vi "Data Server Find Indexes from Variable Names.vi"(8 "Comand string":string, 11 "Variable names":string[](array[string])) -> (0 "Command error":bool, 3 "Index array":i32[](array[numeric]))   [LabVIEW 2011, in "Data Server VIs.lvlib"]
uses:
  Data Server VIs.lvlib
panel:
  in  "Number of BPM":i32
  in  "comand string 2":string="ACH05AACH06ACH07AACH02ACH01B"
  in  "BPM names":string[](array[string])=["ACH01B", "ACH02", "ACH03B", "ACH04", "ACH05A", "ACH06", "ACH07A", "ACH07B", "ACH08"]
  out "Command error 2":bool
  out "Index array 2":i32[](array[numeric])
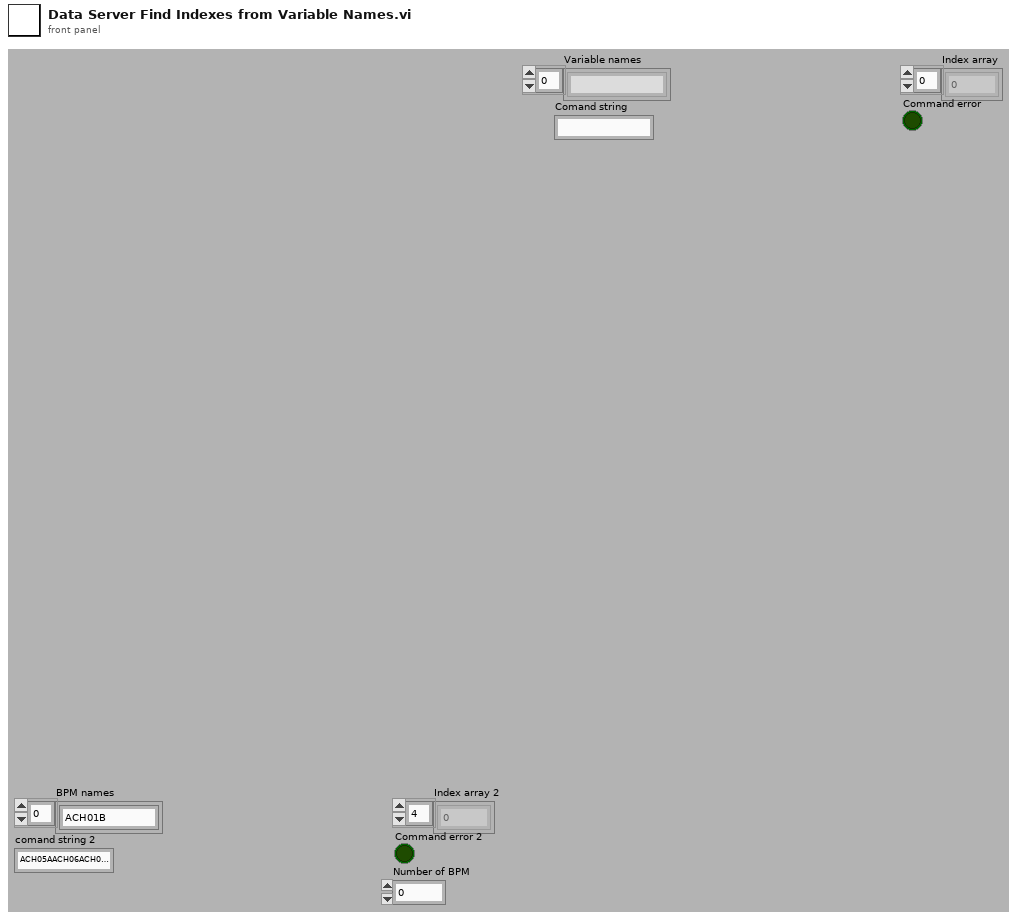
[diagram p1: front panel]
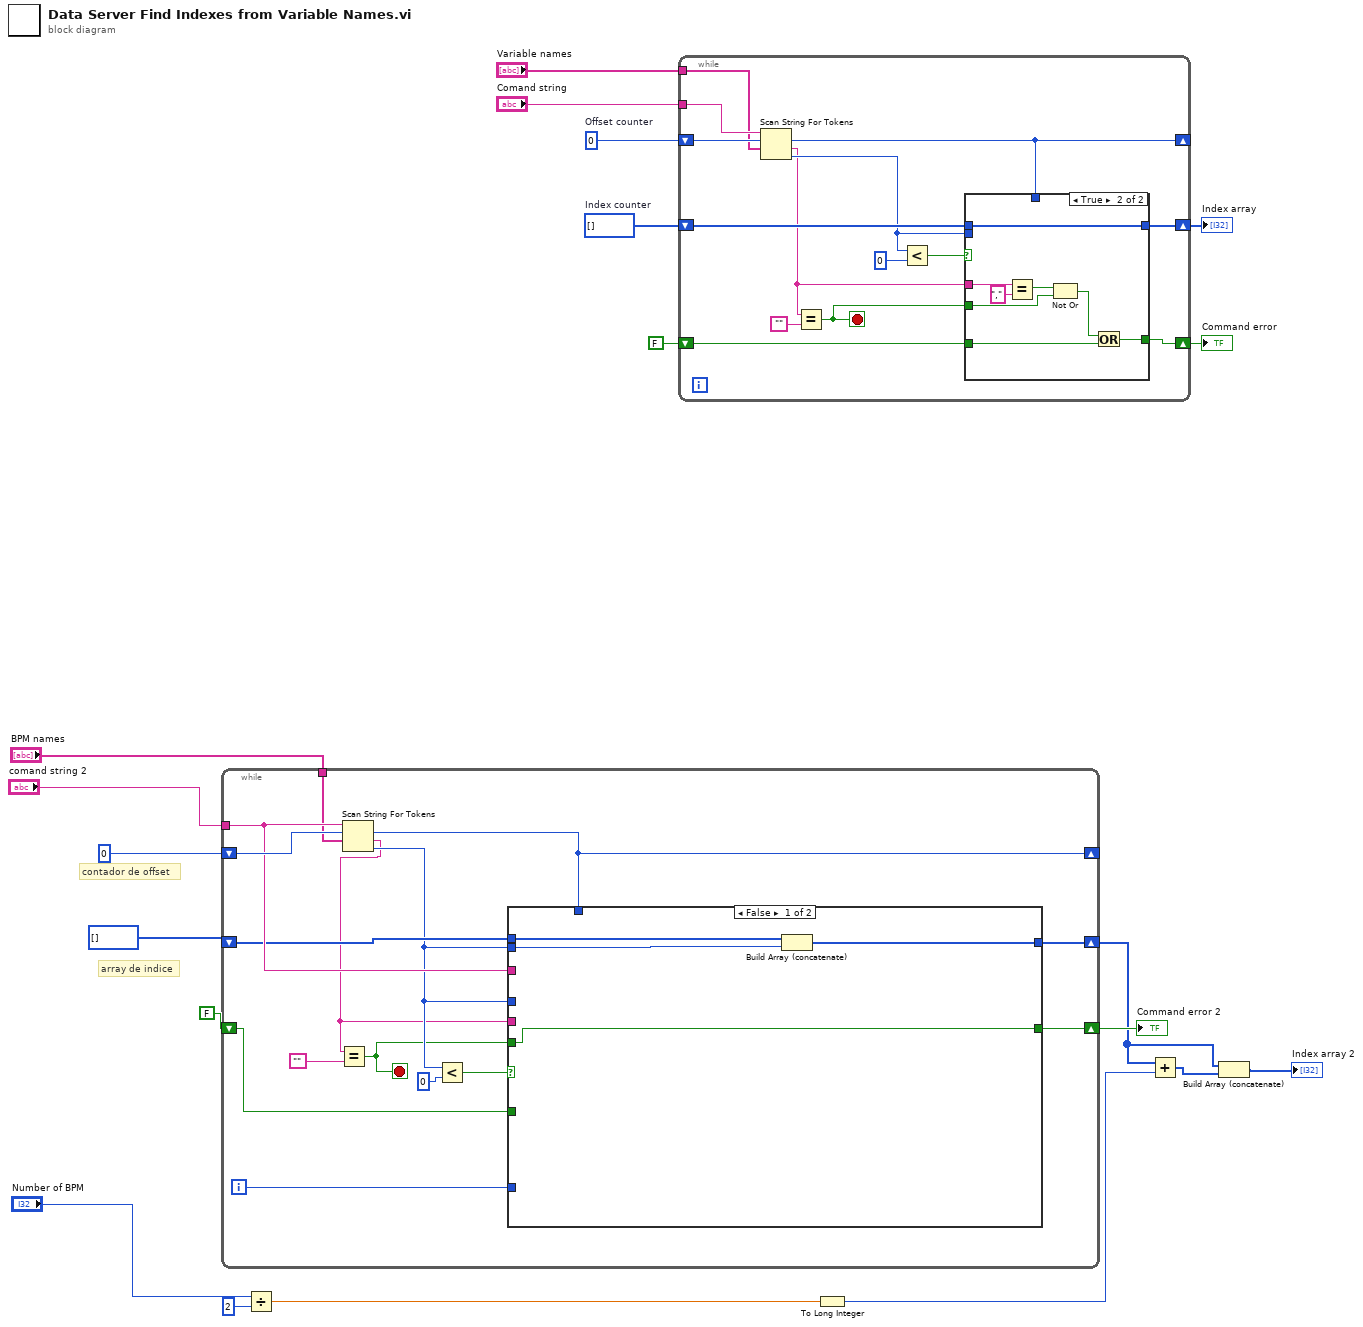
[diagram p0: block diagram]
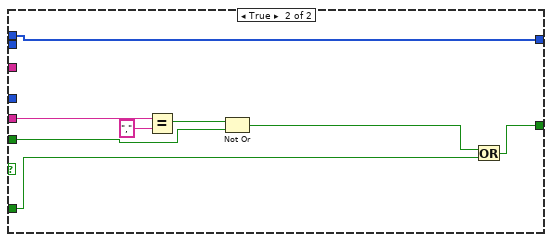
[diagram p2: hidden frame]
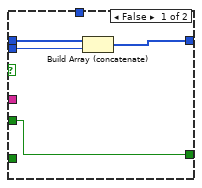
[diagram p3: hidden frame]
diagram:
  w19 = i32[] []  # Index counter
  w20 = 0  # Offset counter
  # "contador de offset"
  # "array de indice"
  n1 = while {
    tunnel: "comand string 2" -> [w30]
    shift-right: [w31] -> _
    shift-left: 0 ("offset past token") -> [w35]
    shift-right: [w28] -> w3
    shift-left: i32[] [] -> [w29]
    tunnel: "BPM names" -> [w26]
    shift-right: [w22] -> w12
    shift-left: FALSE -> [w21]
    i -> [w27]
    stop <- w23 stop-if-true
    n2 = Scan String For Tokens(7:w26, 8:w35, 9:w30) -> (0:w25:i32, 1:w24:string, 2:w31:i32)  [unwired: 3 in, 1 out]
    n3 = Equal?(x=w24, y="") -> (x = y?=w23:bool)
    n4 = Less?(x=w25, y=0) -> (x < y?=w33:bool)
    n5 = case shown="False" w33 {
      tunnel: w25 -> [w38 _]
      tunnel: w31 -> [_ _]
      tunnel: w30 -> [_ _]
      tunnel: w29 -> [w39 w47]
      tunnel: [w37 w47] -> w28
      tunnel: w27 -> [_ _]
      tunnel: w25 -> [_ _]
      tunnel: w24 -> [_ w46]
      tunnel: w23 -> [w36 w43]
      tunnel: [w36 w40] -> w22
      tunnel: w21 -> [_ w42]
      frame False {
        n6 = Build Array (concatenate)(w39, w38) -> (w37:i32[])
      }
      frame True {
        n7 = Equal?(x=w46, y=",") -> (x = y?=w44:bool)
        n8 = Not Or(1:w43, 2:w44) -> (0:w41:bool)
        n9 = Or(x=w41, y=w42) -> (x .or. y?=w40:bool)
      }
    }
  }
  "Command error 2" <- w12
  n10 = Divide(x="Number of BPM", y=2) -> (x/y=w6:dbl)
  n11 = while {
    tunnel: "Comand string" -> [w56]
    shift-right: [w57] -> _
    shift-left: w20 -> [w61]
    shift-right: [w54] -> w15
    shift-left: w19 -> [w55]
    shift-right: [w50] -> w18
    shift-left: FALSE -> [w49]
    tunnel: "Variable names" -> [w48]
    stop <- w51 stop-if-true
    n12 = Scan String For Tokens(7:w48, 8:w61, 9:w56) -> (0:w53:i32, 1:w52:string, 2:w57:i32)  [unwired: 3 in, 1 out]
    n13 = Equal?(x=w52, y="") -> (x = y?=w51:bool)
    n14 = Less?(x=w53, y=0) -> (x < y?=w59:bool)
    n15 = case shown="True" w59 {
      tunnel: w53 -> [w64 _]
      tunnel: w57 -> [_ _]
      tunnel: w55 -> [w65 w73]
      tunnel: [w63 w73] -> w54
      tunnel: w52 -> [_ w72]
      tunnel: w51 -> [w62 w69]
      tunnel: [w62 w66] -> w50
      tunnel: w49 -> [_ w68]
      frame False {
        n16 = Build Array (concatenate)(w65, w64) -> (w63:i32[])
      }
      frame True {
        n17 = Equal?(x=w72, y=",") -> (x = y?=w70:bool)
        n18 = Not Or(1:w69, 2:w70) -> (0:w67:bool)
        n19 = Or(x=w67, y=w68) -> (x .or. y?=w66:bool)
      }
    }
  }
  "Index array" <- w15
  "Command error" <- w18
  n20 = To Long Integer(number=w6) -> (32bit integer=w5:i32)
  n21 = Add(x=w3, y=w5) -> (x+y=w4:i32[])
  n22 = Build Array (concatenate)(w3, w4) -> (→"Index array 2":i32[])
